vi "Read Waveform.vi"(8 "error in (no error)":errorcluster, 11 "NI DMM in":refnum<class "NI DMM.lvclass">) -> (0 "error out":errorcluster, 2 "Data":variant, 3 "NI DMM out":refnum<class "NI DMM.lvclass">)   [LabVIEW 2020, in "NI DMM.lvlib" / "NI DMM.lvclass"]
uses:
  NI DMM.lvclass
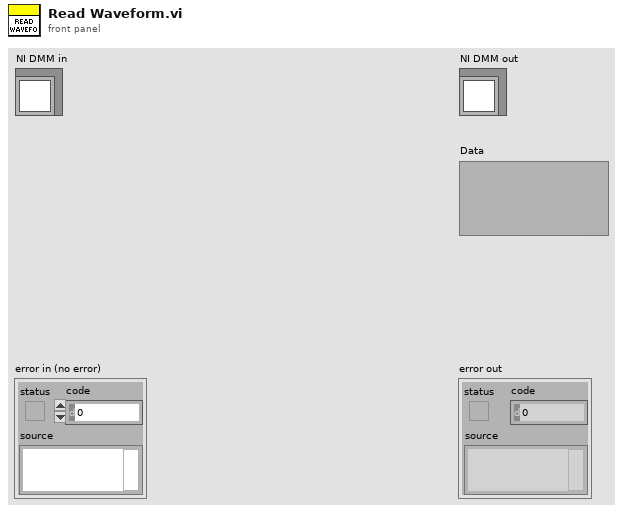
[diagram p1: front panel]
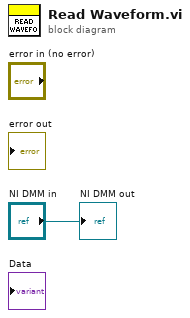
[diagram p0: block diagram]
diagram:
  "NI DMM out" <- "NI DMM in"
